vi "VCI Init CAN.vi"(7 "pInitConfig":T1, 8 "error in (no error)":errorcluster, 9 "CANIndex":u32, 10 "DevIndex":u32, 11 "DevType":u32) -> (0 "error out":errorcluster, 3 "function return":u32)   [LabVIEW 2012, in "ControlCAN.lvlib"]
doc: "unsigned int WINAPI VCI_InitCAN(unsigned int DevType, unsigned int DevIndex, unsigned int CANIndex, PVCI_INIT_CONFIG pInitConfig);"
uses:
  ControlCAN.lvlib
  Ginkgo_Driver.dll
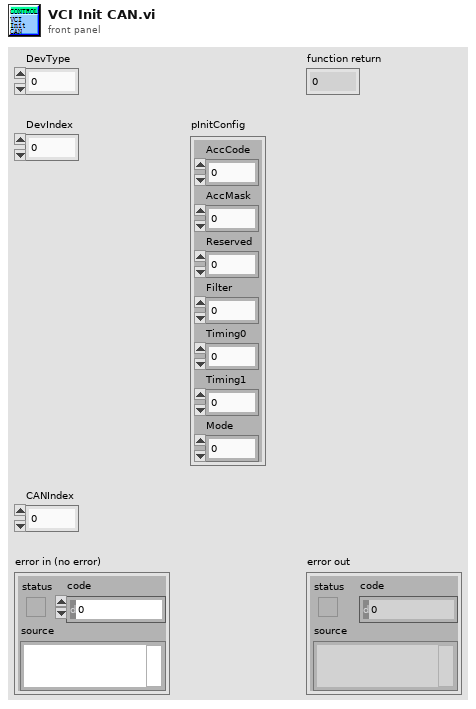
[diagram p1: front panel]
types:
  T1 = cluster{"AccCode":u32, "AccMask":u32, "Reserved":u32, "Filter":u8, "Timing0":u8, "Timing1":u8, "Mode":u8}
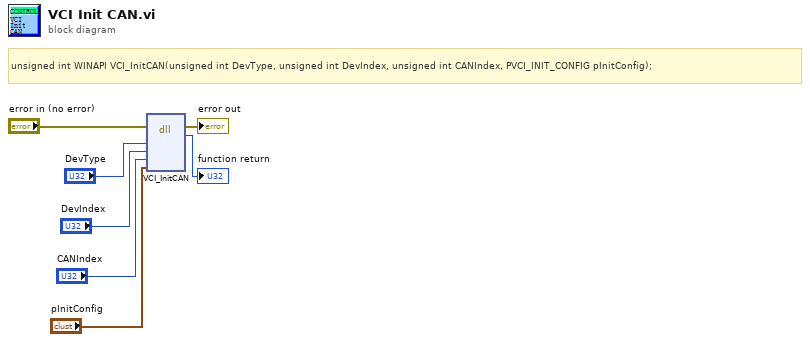
[diagram p0: block diagram]
diagram:
  # "unsigned int WINAPI VCI_InitCAN(unsigned int DevType, unsigned int DevIndex, unsigned int CANIndex, PVCI_INIT_CONFIG pInitConfig);"
  n1 = dll-call lib="E:/Project/vt_ginkgo/truck/Ginkgo Driver/vs2010/Ginkgo_USB-I2C_API_v2.0.3.0/lib/labview_32bit/ControlCAN/Ginkgo_Driver.*" fn="VCI_InitCAN"(error in="error in (no error)", "DevType"="DevType", "DevIndex"="DevIndex", "CANIndex"="CANIndex", "pInitConfig"="pInitConfig") -> (error out=→"error out":errorcluster, →"function return":u32)  [unwired: 6 in, 1 out]
